vi "Create Panel by Type.vi"(7 "Panel Type":refnum<class "ArrayPanel.lvclass">, 8 "error in (no error)":errorcluster, 9 "Run? (T)":bool=TRUE, 11 "PanelArray in":refnum<class "ArrayManager.lvclass">) -> (0 "error out":errorcluster, 2 "Panel":refnum<class "ArrayPanel.lvclass">, 3 "PanelArray out":refnum<class "ArrayManager.lvclass">)   [LabVIEW 2020, in "OOPanel.lvlib" / "ArrayManager.lvclass"]
uses:
  ArrayManager.lvclass
  ArrayPanel/ArrayPanel.lvclass
  C:/dev/LabVIEW/lv-oopanel/OOPanel/Panel/Panel.lvclass
  ArrayManager.lvclass/ArrayManager.ctl
  ArrayPanel/ArrayPanel.lvclass/ArrayPanel.ctl
  Manager/Manager.lvclass
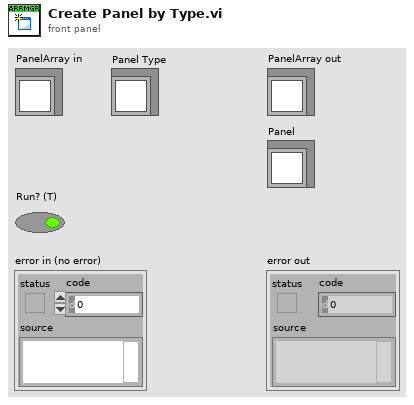
[diagram p1: front panel]
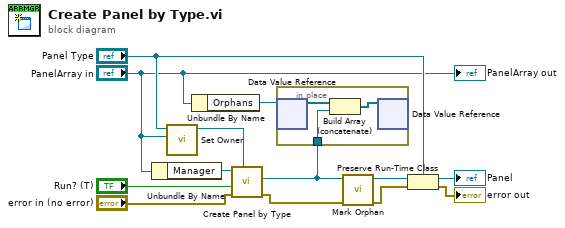
[diagram p0: block diagram]
diagram:
  n1 = Unbundle By Name("PanelArray in") -> ("Manager"=w13:refnum<class "Manager.lvclass">)
  n2 = call "Set Owner.vi"("Owner"="PanelArray in", "ArrayPanel in"="Panel Type") -> ("ArrayPanel out"=w5:refnum<class "ArrayPanel.lvclass">)  [unwired: 8 in, 1 out]
  n3 = Unbundle By Name("PanelArray in") -> ("Orphans"=w8:refnum<data-value>)
  n4 = call "Create Panel by Type.vi"("Panel Type"=w5, "error in (no error)"="error in (no error)", "Run? (T)"="Run? (T)", "Manager in"=w13) -> ("error out"=w1:errorcluster, "Panel"=w2:refnum<class "ArrayPanel.lvclass">)  [unwired: 5 in, 1 out]
  n5 = in-place {
    in-place-border: w2 -> [w15]
    n6 = in-place-dvr #1(w8) -> (w16:refnum<class "ArrayPanel.lvclass">[])  [unwired: 1 out]
    n7 = Build Array (concatenate)(w16, w15) -> (w14:refnum<class "ArrayPanel.lvclass">[])
    n8 = in-place-dvr #1(w14) -> ()  [unwired: 2 out]
  }
  n9 = call "Mark Orphan.vi"("error in (no error)"=w1, "ArrayPanel in"=w2) -> ("error out"=w6:errorcluster, "ArrayPanel out"=w7:refnum<class "ArrayPanel.lvclass">)  [unwired: 8 in]
  n10 = Preserve Run-Time Class(object in=w7, error in=w6, 2:"Panel Type") -> (object out=→"Panel":refnum<class "ArrayPanel.lvclass">, error out=→"error out":errorcluster)
  "PanelArray out" <- "PanelArray in"
